vi "Check Status.vi"(8 "error in (no error)":errorcluster, 11 "Temperature Controller in":refnum<class "Temperature Controller.lvclass">) -> (0 "error out":errorcluster, 1 "Status":string, 2 "Ready?":bool, 3 "Temperature Controller out":refnum<class "Temperature Controller.lvclass">)   [LabVIEW 2009, in "Temperature Controller.lvclass"]
doc: "(Dynamic) Check if the instrument is powered on and update its member fields with the instrument's current status. Optionally return a text status message."
uses:
  Temperature Controller.lvclass
  Temperature Controller.lvclass/Temperature Controller.ctl
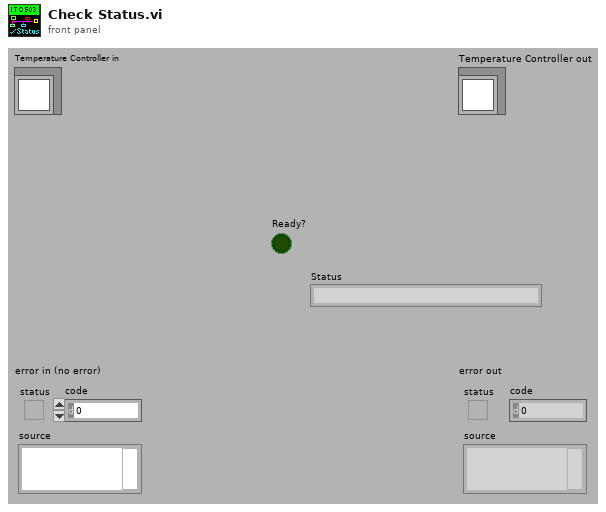
[diagram p1: front panel]
types:
  T1 = typedef "OxfordAddress.ctl" = cluster{"Com Port":i32, "ISOBUS Address":i32, "GPIB Address":i16, "Communication":enum16{"RS232", "ISOBUS", "GPIB", "Gateway"}}
  T2 = typedef "Temperature Controller.lvclass/HV Slide Indicator.ctl" = dbl
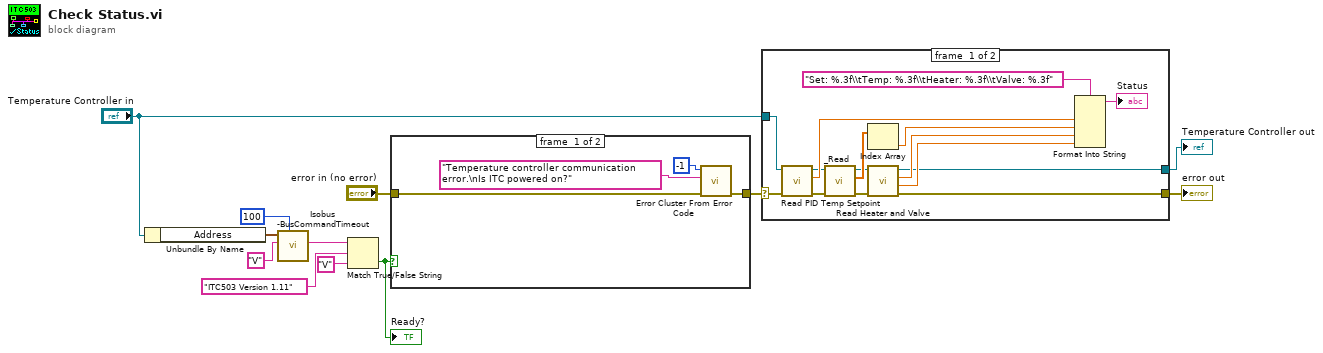
[diagram p0: block diagram]
diagram:
  n1 = Unbundle By Name("Temperature Controller in") -> ("Address"=w3:T1)
  n2 = call "Isobus -BusCommandTimeout.vi"("Timeout (ms)"=100, "Command"="V", "Address"=w3) -> ("Reply"=w1:string)  [unwired: 5 out]
  n3 = Match True/False String(2:"V", 3:"ITC503 Version 1.11", 4:w1) -> (0:w5:bool)  [unwired: 1 out]
  "Ready?" <- w5
  n4 = case shown="False" w5 {
    tunnel: "error in (no error)" -> [w14 w17]
    tunnel: [w13 w17] -> w9
    frame #0 {
      n5 = call <vilib>:"Error Cluster From Error Code.vi"("error in (no error)"=w14, "error message (\"\")"="Temperature controller communication error.\nIs ITC powered on?" ("error message (\"\")"), "error code (0)"=-1) -> ("error out"=w13:errorcluster)  [unwired: 6 in]
    }
    frame #1 {
    }
  }
  n6 = case shown="No Error" w9 {
    selector: w9 -> [w23 w34]
    tunnel: [w18 w33] -> w12
    tunnel: "Temperature Controller in" -> [w22 w33]
    tunnel: [w19 w34] -> w11
    frame #0 {
      n7 = call-dynamic "Read PID Temp Setpoint.vi"("error in (no error)"=w23, "Temperature Controller in"=w22) -> ("error out"=w20:errorcluster, "PID Temp Setpoint"=w24:dbl[unit], "Temperature Controller out"=w21:refnum<class "Temperature Controller.lvclass">)  [unwired: 7 in]
      n8 = call-dynamic "_Read.vi"("error in (no error)"=w20, "Temperature Controller.lvclass"=w21) -> ("error out"=w26:errorcluster, "Data Points"=w30:dbl[], "Temperature Controller out"=w29:refnum<class "Temperature Controller.lvclass">)  [unwired: 7 in]
      n9 = Index Array(array=w30) -> (element=w25:dbl)  [unwired: 1 in]
      n10 = call-dynamic "Read Heater and Valve.vi"("error in (no error)"=w26, "Temperature Controller in"=w29) -> ("error out"=w19:errorcluster, "valve%"=w27:T2, "heater%"=w28:T2, "Temperature Controller out"=w18:refnum<class "Temperature Controller.lvclass">)  [unwired: 6 in]
      n11 = Format Into String(format string="Set: %.3f\\tTemp: %.3f\\tHeater: %.3f\\tValve: %.3f", w24, w25, w28, w27) -> (resulting string=→"Status":string)  [unwired: 2 in, 1 out]
    }
    frame #1 {
    }
  }
  "error out" <- w11
  "Temperature Controller out" <- w12
